vi "Main.vi"() -> ()   [LabVIEW 2021]
uses:
  controls/UI Data.ctl
  controls/ID.ctl
  controls/TCP states.ctl
  169f6d76-e22e-422a-8878-d2a9cb751e73.vi
  6a9415bc-3281-45d9-a9d8-b5f40684fea4.vi
  904bcb0e-ec7b-4b25-8705-34aa29b38f14.vi
  fb36bc3e-c328-4c18-9bea-3fff38157571.vi
  34653ac8-04e4-4dac-97e9-0b17219b7a3c.vi
  4f2ca51b-55f9-45ce-8b7e-e77bf4893014.vi
  ef0f1724-a7e1-494b-ab43-6d28ffb4e330.vi
  49fa5557-646f-45f4-af6f-6dd531291f5f.vi
  d94f9ece-38ec-4846-8ebf-07454e2bacb2.vi
panel:
  out "Response":string
  out "DS":bool
  out "WA":bool
  out "WC":bool
  in  "Stop":bool
  in  "My App path":path=path "c:/My App"
  in  "Reboot":bool
  out "PWR":bool
  out "WS":bool
  out "DC":bool
  out "SM":bool
  out "Commands":string[][](array[string])
  in  "Config path":path=path "C:/Users/ken_X/Documents/LabVIEW projects/Project-B/settings/config.xls"
  in  "Version path":path=path "C:/4.9.12.6034"
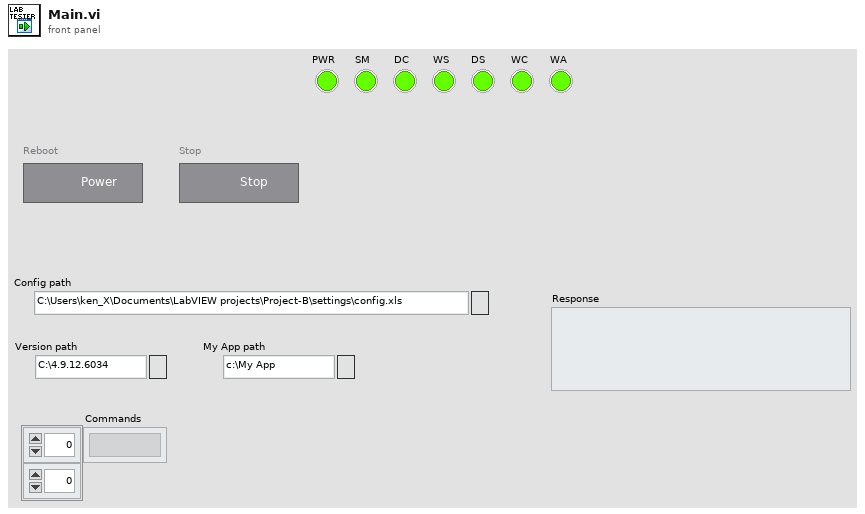
[diagram p1: front panel]
types:
  T1 = typedef "UI Data.ctl" = cluster{"Config path":path, "Version path":path, "My App path":path, "Racks":u16}
  T2 = cluster{"accent s color":u32, "accent s color":u32}
  T3 = typedef "ID.ctl" = enum16{"1 - PWR", "2 - SM", "3 - DC", "4 - DM", "5 - WS", "6 - DS", "7 - WC", "8 - WA", "9 - WM", "10 - DA", "11 - WH", "12 - DH"}
  T4 = typedef "TCP states.ctl" = string
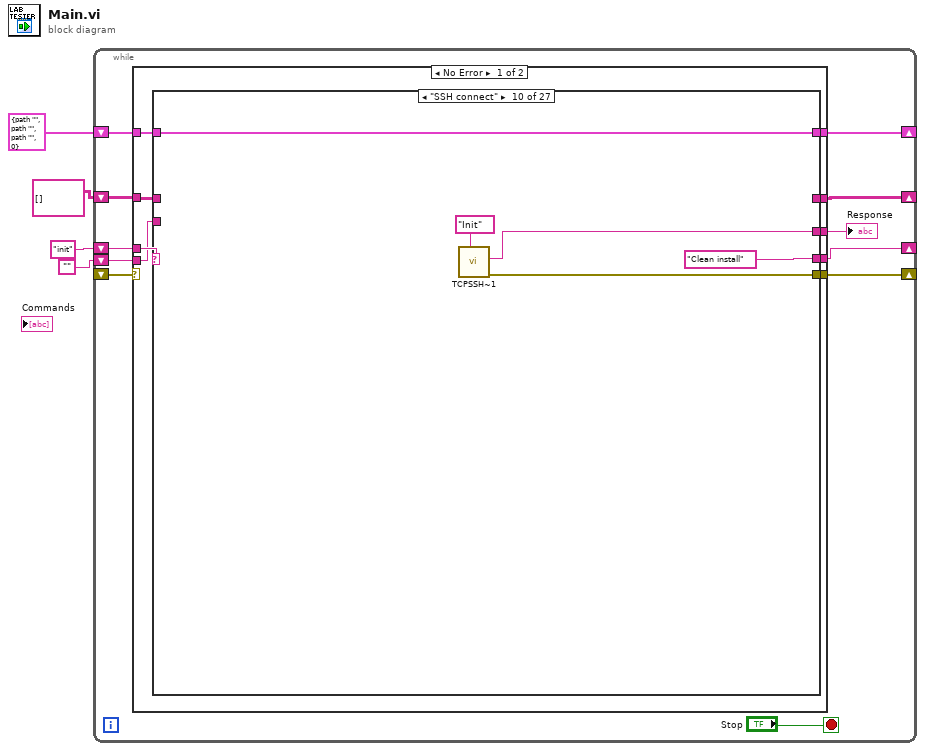
[diagram p0: block diagram]
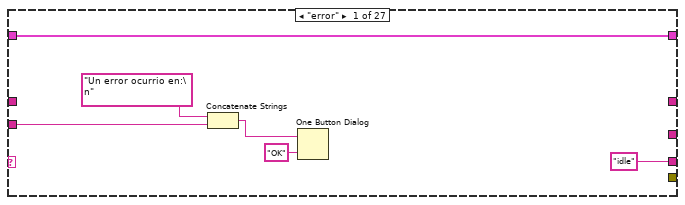
[diagram p2: hidden frame]
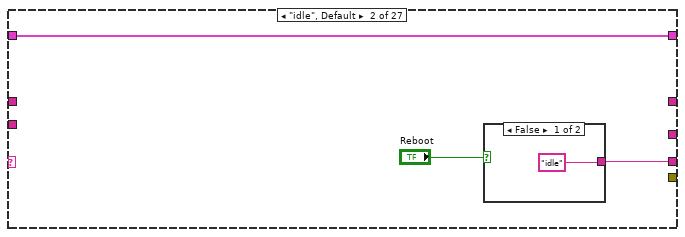
[diagram p3: hidden frame]
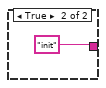
[diagram p4: hidden frame]
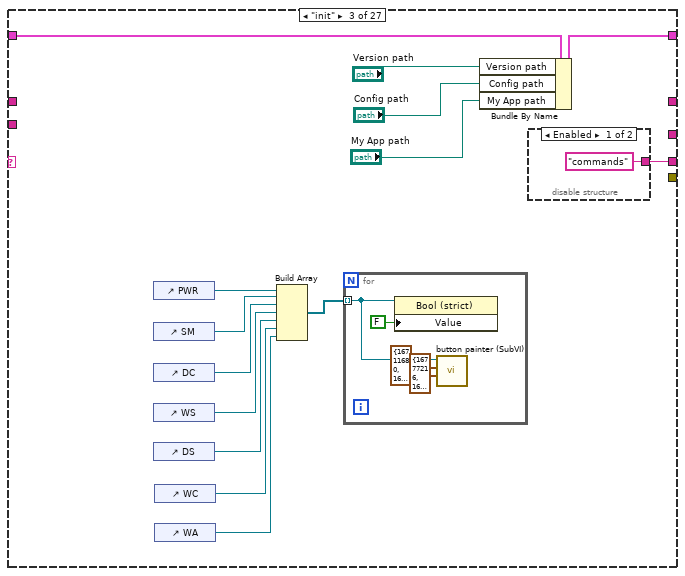
[diagram p5: hidden frame]
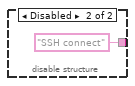
[diagram p6: hidden frame]
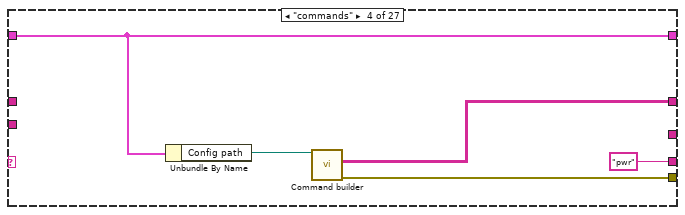
[diagram p7: hidden frame]
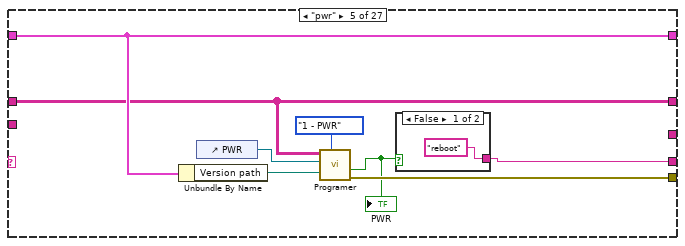
[diagram p8: hidden frame]
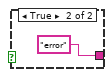
[diagram p9: hidden frame]
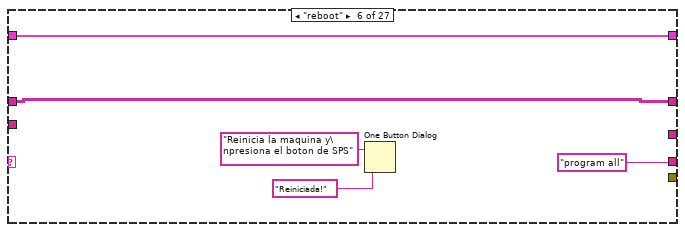
[diagram p10: hidden frame]
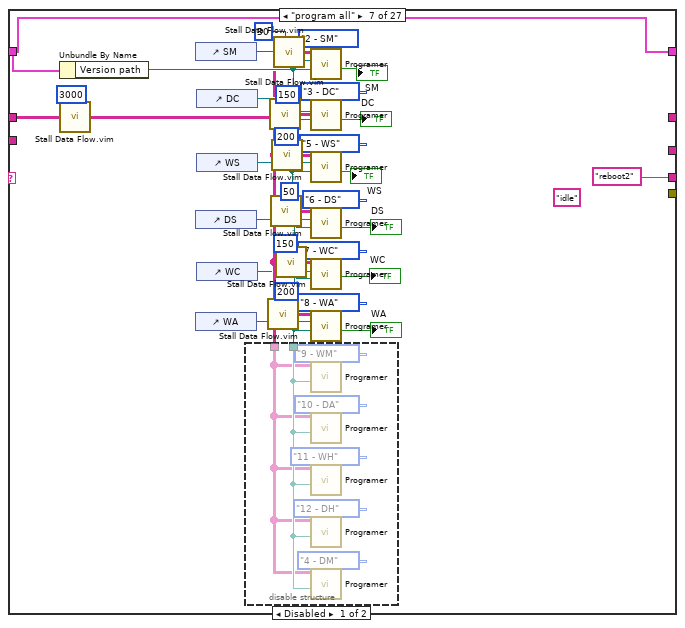
[diagram p11: hidden frame]
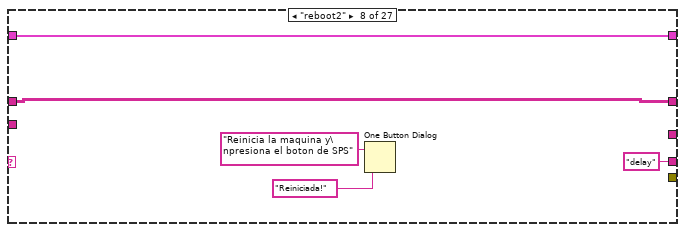
[diagram p13: hidden frame]
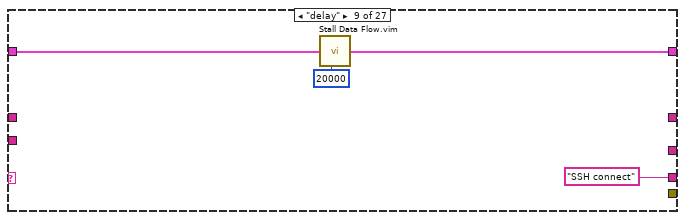
[diagram p14: hidden frame]
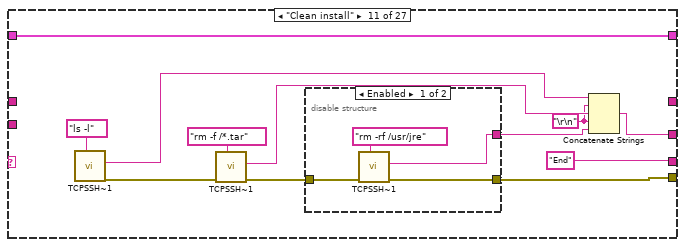
[diagram p15: hidden frame]
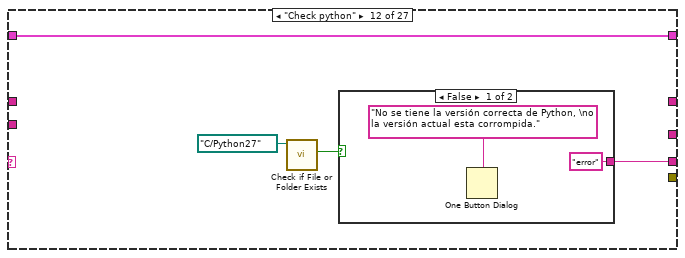
[diagram p17: hidden frame]
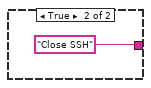
[diagram p18: hidden frame]
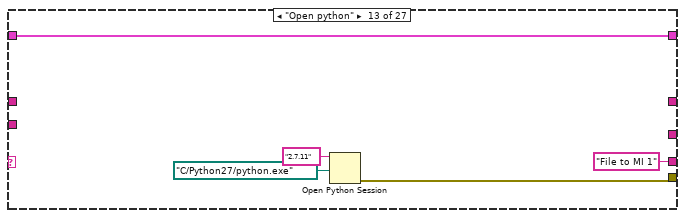
[diagram p19: hidden frame]
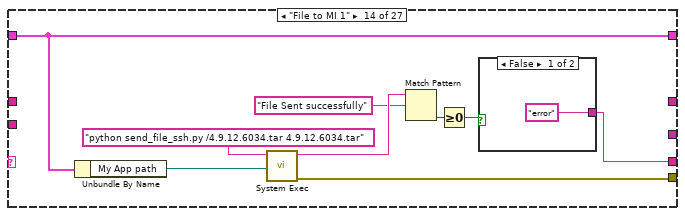
[diagram p20: hidden frame]
diagram:
  n1 = while {
    shift-right: [w13] -> _
    shift-left: T1 {"Config path"=path "", "Version path"=path "", "My App path"=path "", "Racks"=0} ("Cluster") -> [w14]
    shift-right: [w12] -> _
    shift-left: "init" -> [w15]
    shift-right: [w11] -> _
    shift-left: _ -> [w10]
    shift-right: [w9] -> _
    shift-left: string[][] [] ("Commands") -> [w8]
    shift-left: "" -> [w7]
    stop <- "Stop" stop-if-true
    n2 = case shown="No Error" w10 {
      selector: w10 -> [_ w296]
      tunnel: w15 -> [w24 _]
      tunnel: w14 -> [w23 _]
      tunnel: [w22 _] -> w13
      tunnel: [w21 "idle"] -> w12
      tunnel: [w20 _] -> w11
      tunnel: [w19 _] -> w9
      tunnel: w8 -> [w18 _]
      tunnel: w7 -> [w17 w295]
      tunnel: [w16 _] -> w5
      frame No Error {
        n3 = case shown="\"SSH connect\"" w24 {
          tunnel: w23 -> [w25 w33 w49 w57 w67 w71 w110 w120 w127 w129 w141 w153 w161 w164 w175 w189 w203 w207 w212 w227 w231 w241 w253 w259 w266 w290 w293]
          tunnel: [w25 w33 w48 w57 w67 w71 w110 w120 w125 w129 w141 w153 w161 w164 w175 w189 w203 w207 w212 w227 w231 w241 w253 w259 w265 w290 w293] -> w22
          tunnel: ["idle" w31 w47 "pwr" w62 "program all" "reboot2" "delay" "SSH connect" "Clean install" "End" w150 "File to MI 1" w165 w173 "Kill all" "Copy rootfs" "Sync" w208 "Telnet" "Search Data" w232 w244 "Check racks" w260 "End" "idle"] -> w21
          tunnel: [_ _ _ w60 w66 _ _ _ _ w131 w142 _ w158 w162 w177 w185 w192 w205 w209 w221 w229 w233 w245 w257 w263 w289 _] -> w20
          tunnel: [_ _ _ w58 w65 w72 _ w121 _ _ _ _ _ _ _ _ _ _ _ _ _ _ _ _ _ _ _] -> w19
          tunnel: w18 -> [_ _ _ _ w65 w72 w107 w121 _ _ _ _ _ _ _ _ _ _ _ _ _ _ _ _ _ _ _]
          tunnel: w17 -> [w29 _ _ _ _ _ _ _ _ _ _ _ _ _ _ _ _ _ _ _ _ _ _ _ _ _ _]
          tunnel: [_ _ _ _ _ _ _ _ _ w128 w138 _ _ _ _ _ _ _ _ _ _ _ _ _ _ _ _] -> w16
          frame "error" {
            n4 = Concatenate Strings("Un error ocurrio en:\n" ("string"), w29) -> (w28:string)
            n5 = One Button Dialog(message=w28, button name ("OK")="OK") -> ()  [unwired: 1 out]
          }
          frame "idle", Default {
            n6 = case shown="False" "Reboot" {
              tunnel: ["idle" "init"] -> w31
              frame False {
              }
              frame True {
              }
            }
          }
          frame "init" {
            n7 = control-ref of="PWR"() -> (w43:refnum<vi>)
            n8 = control-ref of="SM"() -> (w42:refnum<vi>)
            n9 = control-ref of="DC"() -> (w41:refnum<vi>)
            n10 = control-ref of="WS"() -> (w40:refnum<vi>)
            n11 = control-ref of="DS"() -> (w38:refnum<vi>)
            n12 = control-ref of="WC"() -> (w37:refnum<vi>)
            n13 = control-ref of="WA"() -> (w36:refnum<vi>)
            n14 = Build Array(w43, w42, w41, w40, w38, w37, w36) -> (w39:refnum<vi>[])
            n15 = for {
              tunnel: w39 -> [w54] mode=indexing
              n16 = property class="Bool (strict)"(reference=w54, "Value"=FALSE) -> ()  [unwired: 1 in, 2 out]
              n17 = call "button painter (SubVI).vi"("Off state"=cluster{"accent color":u32, "accent color":u32} {"accent color"=16777216, "accent color"=16777216}, "On state"=T2 {"accent s color"=16711680, "accent s color"=16711680}, "Button ref in"=w54) -> ()  [unwired: 9 in]
            }
            n18 = Bundle By Name(cluster=w49, "Version path"="Version path", "Config path"="Config path", "My App path"="My App path") -> (w48:T1)
            n19 = disable-structure shown="Enabled" {
              disable-tunnel: ["commands" "SSH connect"] -> w47
              frame Enabled {
              }
              frame Disabled {
              }
            }
          }
          frame "commands" {
            n20 = Unbundle By Name(w57) -> ("Config path"=w56:path)
            n21 = call "Command builder.vi"("Config path"=w56) -> ("error out"=w60:errorcluster, "Commands"=w58:string[][])  [unwired: 9 in]
          }
          frame "pwr" {
            n22 = Unbundle By Name(w67) -> ("Version path"=w63:path)
            n23 = control-ref of="PWR"() -> (w61:refnum<vi>)
            n24 = call "Programer.vi"("ID"=ID."1 - PWR", "version path"=w63, "Bool Ref"=w61, "Commands"=w65) -> ("error out"=w66:errorcluster, "error?"=w64:bool)  [unwired: 5 in, 1 out]
            "PWR" <- w64
            n25 = case shown="False" w64 {
              tunnel: ["reboot" "error"] -> w62
              frame False {
              }
              frame True {
              }
            }
          }
          frame "reboot" {
            n26 = One Button Dialog(message="Reinicia la maquina y\npresiona el boton de SPS", button name ("OK")="Reiniciada!") -> ()  [unwired: 1 out]
          }
          frame "program all" {
            (unwired) "idle"
            n27 = Unbundle By Name(w110) -> ("Version path"=w105:path)
            n28 = call "Stall Data Flow.vim"("value in"=w107, "milliseconds to wait"=u32 3000) -> ("value out"=w97:string[][])  [unwired: 1 out]
            n29 = control-ref of="SM"() -> (w104:refnum<vi>)
            n30 = control-ref of="DS"() -> (w92:refnum<vi>)
            n31 = control-ref of="WA"() -> (w90:refnum<vi>)
            n32 = control-ref of="DC"() -> (w103:refnum<vi>)
            n33 = control-ref of="WS"() -> (w102:refnum<vi>)
            n34 = control-ref of="WC"() -> (w91:refnum<vi>)
            n35 = disable-structure shown="Disabled" {
              disable-tunnel: w105 -> [w118 _]
              disable-tunnel: w97 -> [w117 _]
              frame Disabled {
                n36 = call "Programer.vi"("ID"=ID."9 - WM", "version path"=w118, "Commands"=w117) -> ()  [unwired: 6 in, 3 out]
                n37 = call "Programer.vi"("ID"=ID."10 - DA", "version path"=w118, "Commands"=w117) -> ()  [unwired: 6 in, 3 out]
                n38 = call "Programer.vi"("ID"=ID."11 - WH", "version path"=w118, "Commands"=w117) -> ()  [unwired: 6 in, 3 out]
                n39 = call "Programer.vi"("ID"=ID."12 - DH", "version path"=w118, "Commands"=w117) -> ()  [unwired: 6 in, 3 out]
                n40 = call "Programer.vi"("ID"=ID."4 - DM", "version path"=w118, "Commands"=w117) -> ()  [unwired: 6 in, 3 out]
              }
              frame Enabled {
              }
            }
            n41 = call "Stall Data Flow.vim"("value in"=w97, "milliseconds to wait"=u32 200) -> ("value out"=w78:string[][])  [unwired: 1 out]
            n42 = call "Stall Data Flow.vim"("value in"=w97, "milliseconds to wait"=u32 150) -> ("value out"=w86:string[][])  [unwired: 1 out]
            n43 = call "Stall Data Flow.vim"("value in"=w97, "milliseconds to wait"=u32 50) -> ("value out"=w82:string[][])  [unwired: 1 out]
            n44 = call "Stall Data Flow.vim"("value in"=w97, "milliseconds to wait"=u32 200) -> ("value out"=w84:string[][])  [unwired: 1 out]
            n45 = call "Stall Data Flow.vim"("value in"=w97, "milliseconds to wait"=u32 50) -> ("value out"=w99:string[][])  [unwired: 1 out]
            n46 = call "Stall Data Flow.vim"("value in"=w97, "milliseconds to wait"=u32 150) -> ("value out"=w80:string[][])  [unwired: 1 out]
            n47 = call "Programer.vi"("ID"=ID."2 - SM", "version path"=w105, "Bool Ref"=w104, "Commands"=w99) -> ("error?"=→"SM":bool)  [unwired: 5 in, 2 out]
            n48 = call "Programer.vi"("ID"=ID."3 - DC", "version path"=w105, "Bool Ref"=w103, "Commands"=w86) -> ("error?"=→"DC":bool)  [unwired: 5 in, 2 out]
            n49 = call "Programer.vi"("ID"=ID."5 - WS", "version path"=w105, "Bool Ref"=w102, "Commands"=w84) -> ("error?"=→"WS":bool)  [unwired: 5 in, 2 out]
            n50 = call "Programer.vi"("ID"=ID."6 - DS", "version path"=w105, "Bool Ref"=w92, "Commands"=w82) -> ("error?"=→"DS":bool)  [unwired: 5 in, 2 out]
            n51 = call "Programer.vi"("ID"=ID."7 - WC", "version path"=w105, "Bool Ref"=w91, "Commands"=w80) -> ("error?"=→"WC":bool)  [unwired: 5 in, 2 out]
            n52 = call "Programer.vi"("ID"=ID."8 - WA", "version path"=w105, "Bool Ref"=w90, "Commands"=w78) -> ("error?"=→"WA":bool)  [unwired: 5 in, 2 out]
          }
          frame "reboot2" {
            n53 = One Button Dialog(message="Reinicia la maquina y\npresiona el boton de SPS", button name ("OK")="Reiniciada!") -> ()  [unwired: 1 out]
          }
          frame "delay" {
            n54 = call "Stall Data Flow.vim"("value in"=w127, "milliseconds to wait"=u32 20000) -> ("value out"=w125:T1)  [unwired: 1 out]
          }
          frame "SSH connect" {
            n55 = call "TCPSSH~1.VI"("States"=T4 "Init") -> ("Error  Out"=w131:errorcluster, "Response"=w128:string)  [unwired: 8 in]
          }
          frame "Clean install" {
            w134 = "\r\n"
            n56 = call "TCPSSH~1.VI"("States"=T4 "ls -l") -> ("Error  Out"=w135:errorcluster, "Response"=w133:string)  [unwired: 8 in]
            n57 = call "TCPSSH~1.VI"("States"=T4 "rm -f /*.tar", "Error In"=w135) -> ("Error  Out"=w144:errorcluster, "Response"=w140:string)  [unwired: 7 in]
            n58 = disable-structure shown="Enabled" {
              disable-tunnel: w144 -> [w148 w149]
              disable-tunnel: [w146 w149] -> w142
              disable-tunnel: [w145 _] -> w139
              frame Enabled {
                n59 = call "TCPSSH~1.VI"("States"=T4 "rm -rf /usr/jre", "Error In"=w148) -> ("Error  Out"=w146:errorcluster, "Response"=w145:string)  [unwired: 7 in]
              }
              frame Disabled {
              }
            }
            n60 = Concatenate Strings(w133, w134, w140, w134, w139) -> (w138:string)
          }
          frame "Check python" {
            n61 = call <vilib>:"Check if File or Folder Exists.vi"("path"=path "C:/Python27") -> ("file or folder exists?"=w151:bool)  [unwired: 8 in, 2 out]
            n62 = case shown="False" w151 {
              tunnel: ["error" "Close SSH"] -> w150
              frame False {
                n63 = One Button Dialog(message="No se tiene la versión correcta de Python, \no la versión actual esta corrompida.") -> ()  [unwired: 1 in, 1 out]
              }
              frame True {
              }
            }
          }
          frame "Open python" {
            n64 = Open Python Session(python version="2.7.11" ("Python version"), python path=path "C:/Python27/python.exe" ("Python path")) -> (error out=w158:errorcluster)  [unwired: 1 in, 1 out]
          }
          frame "File to MI 1" {
            n65 = Unbundle By Name(w164) -> ("My App path"=w163:path)
            n66 = call <vilib>:"System Exec.vi"("working directory"=w163, "command line"="python send_file_ssh.py /4.9.12.6034.tar 4.9.12.6034.tar") -> ("error out"=w162:errorcluster, "standard output"=w169:string)  [unwired: 6 in, 2 out]
            n67 = Match Pattern(string=w169, regular expression="File Sent successfully") -> (offset past match=w167:i32)  [unwired: 1 in, 3 out]
            n68 = Greater Or Equal To 0?(x=w167) -> (x >= 0?=w166:bool)
            n69 = case shown="False" w166 {
              tunnel: ["error" "End"] -> w165
              frame False {
              }
              frame True {
                (unwired) "File to MI 2"
              }
            }
          }
          frame "File to MI 2" {
            n70 = Unbundle By Name(w175) -> ("My App path"=w174:path)
            n71 = call <vilib>:"System Exec.vi"("working directory"=w174, "command line"="send_file_to_MI_ssh.bat /jre.tar.gz jre.tar.gz") -> ("error out"=w177:errorcluster, "standard output"=w181:string)  [unwired: 6 in, 2 out]
            n72 = Match Pattern(string=w181, regular expression="File Sent successfully") -> (offset past match=w179:i32)  [unwired: 1 in, 3 out]
            n73 = Greater Or Equal To 0?(x=w179) -> (x >= 0?=w178:bool)
            n74 = case shown="True" w178 {
              tunnel: ["error" "Send tars"] -> w173
              frame False {
              }
              frame True {
              }
            }
          }
          frame "Send tars" {
            n75 = call "TCPSSH~1.VI"("States"=T4 "tar -xvf 4.9.12.6034.tar") -> ("Error  Out"=w188:errorcluster)  [unwired: 8 in, 1 out]
            n76 = call "TCPSSH~1.VI"("States"=T4 "tar -xvf jre.tar.gz -C /usr", "Error In"=w188) -> ("Error  Out"=w185:errorcluster)  [unwired: 7 in, 1 out]
          }
          frame "Kill all" {
            n77 = call "TCPSSH~1.VI"("States"=T4 "rm -f /*.tar") -> ("Error  Out"=w194:errorcluster)  [unwired: 8 in, 1 out]
            n78 = call "TCPSSH~1.VI"("States"=T4 "rm -f /*.gz", "Error In"=w194) -> ("Error  Out"=w196:errorcluster)  [unwired: 7 in, 1 out]
            n79 = call "TCPSSH~1.VI"("States"=T4 "killall DataProcessor.exe", "Error In"=w196) -> ("Error  Out"=w197:errorcluster)  [unwired: 7 in, 1 out]
            n80 = call "TCPSSH~1.VI"("States"=T4 "killall WIFIAgent.exe", "Error In"=w197) -> ("Error  Out"=w199:errorcluster)  [unwired: 7 in, 1 out]
            n81 = call "TCPSSH~1.VI"("States"=T4 "killall java", "Error In"=w199) -> ("Error  Out"=w201:errorcluster)  [unwired: 7 in, 1 out]
            n82 = call "TCPSSH~1.VI"("States"=T4 "killall MonitorDaemon.exe", "Error In"=w201) -> ("Error  Out"=w192:errorcluster)  [unwired: 7 in, 1 out]
          }
          frame "Copy rootfs" {
            n83 = call "TCPSSH~1.VI"("States"=T4 "cp -rf rootfs/* /") -> ("Error  Out"=w205:errorcluster)  [unwired: 8 in, 1 out]
          }
          frame "Sync" {
            n84 = flat-sequence {
              tunnel: [w213] -> w211
              tunnel: w211 -> [w217]
              tunnel: [w216] -> w210
              tunnel: [w219] -> w209
              tunnel: w210 -> [w219]
              tunnel: ["SED"] -> w208
              frame #0 {
                n85 = call "TCPSSH~1.VI"("States"=T4 "sync") -> ("Error  Out"=w213:errorcluster)  [unwired: 8 in, 1 out]
              }
              frame #1 {
                n86 = call "Stall Data Flow.vim"("value in"=w217, "milliseconds to wait"=u32 3000) -> ("value out"=w216:errorcluster)  [unwired: 1 out]
              }
              frame #2 {
              }
            }
          }
          frame "SED" {
            n87 = call "TCPSSH~1.VI"("States"=T4 "cd hdplus") -> ("Error  Out"=w224:errorcluster)  [unwired: 8 in, 1 out]
            n88 = call "TCPSSH~1.VI"("States"=T4 "sed -i", "Error In"=w224) -> ("Error  Out"=w226:errorcluster)  [unwired: 7 in, 1 out]
            n89 = call "TCPSSH~1.VI"("States"=T4 "cat /hdplus/tablo.conf", "Error In"=w226) -> ("Error  Out"=w221:errorcluster)  [unwired: 7 in, 1 out]
          }
          frame "Telnet" {
            n90 = call "TCPSSH~1.VI"("States"=T4 "script/disableTelnet") -> ("Error  Out"=w229:errorcluster)  [unwired: 8 in, 1 out]
          }
          frame "Search Data" {
            n91 = call "TCPSSH~1.VI"("States"=T4 "ls -l") -> ("Error  Out"=w235:errorcluster)  [unwired: 8 in, 1 out]
            n92 = call "TCPSSH~1.VI"("States"=T4 "Read", "Error In"=w235) -> ("Error  Out"=w233:errorcluster, "Response"=w240:string)  [unwired: 7 in]
            n93 = Match Pattern(string=w240, regular expression="DataProcessor.exe") -> (offset past match=w237:i32)  [unwired: 1 in, 3 out]
            n94 = Greater Or Equal To 0?(x=w237) -> (x >= 0?=w238:bool)
            n95 = case shown="True" w238 {
              tunnel: ["error" "Search Java"] -> w232
              frame False {
              }
              frame True {
              }
            }
          }
          frame "Search Java" {
            n96 = call "TCPSSH~1.VI"("States"=T4 "/usr/jre/bin/java -version") -> ("Error  Out"=w247:errorcluster)  [unwired: 8 in, 1 out]
            n97 = call "TCPSSH~1.VI"("States"=T4 "Read", "Error In"=w247) -> ("Error  Out"=w245:errorcluster, "Response"=w252:string)  [unwired: 7 in]
            n98 = Match Pattern(string=w252, regular expression="1.8.0-b132") -> (offset past match=w249:i32)  [unwired: 1 in, 3 out]
            n99 = Greater Or Equal To 0?(x=w249) -> (x >= 0?=w250:bool)
            n100 = case shown="True" w250 {
              tunnel: ["error" "Dev"] -> w244
              frame False {
              }
              frame True {
              }
            }
          }
          frame "Dev" {
            n101 = call "TCPSSH~1.VI"("States"=T4 "cd /dev") -> ("Error  Out"=w257:errorcluster)  [unwired: 8 in, 1 out]
          }
          frame "Check racks" {
            n102 = Unbundle By Name(w266) -> ("Racks"=w261:u16)
            n103 = Equal To 0?(x=w261) -> (x = 0?=w262:bool)
            n104 = case shown="False" w262 {
              tunnel: w261 -> [w274 w285]
              tunnel: [w273 w285] -> w264
              tunnel: [w268 _] -> w263
              tunnel: [w267 "End"] -> w260
              frame False {
                n105 = call "TCPSSH~1.VI"("States"=T4 "ls sd* -l") -> ("Error  Out"=w272:errorcluster)  [unwired: 8 in, 1 out]
                n106 = call "TCPSSH~1.VI"("States"=T4 "Read", "Error In"=w272) -> ("Error  Out"=w268:errorcluster, "Response"=w269:string)  [unwired: 7 in]
                n107 = call "string pattern counter.vi"("pattern"="root", "string"=w269) -> ("Numeric"=w277:i32)  [unwired: 9 in]
                n108 = Multiply(x=w274, y=2) -> (x*y=w281:i32)
                n109 = Equal?(x=w281, y=w277) -> (x = y?=w276:bool)
                n110 = Format Into String(format string="Quite una de las %d unidades montadas", w274) -> (resulting string=w275:string)  [unwired: 2 in, 1 out]
                n111 = case shown="True" w276 {
                  tunnel: w275 -> [_ w284]
                  tunnel: ["error" "Check racks"] -> w267
                  frame False {
                  }
                  frame True {
                    n112 = One Button Dialog(message=w284) -> ()  [unwired: 1 in, 1 out]
                  }
                }
                n113 = Decrement(x=w274) -> (x-1=w273:u16)
              }
              frame True {
              }
            }
            n114 = Bundle By Name(cluster=w266, "Racks"=w264) -> (w265:T1)
          }
          frame "Close SSH" {
            n115 = call "TCPSSH~1.VI"("States"=T4 "Close") -> ("Error  Out"=w289:errorcluster)  [unwired: 8 in, 1 out]
          }
          frame "End" {
            n116 = One Button Dialog(message="Proceso terminado!!!") -> ()  [unwired: 1 in, 1 out]
          }
        }
      }
      frame Error {
        n117 = call <vilib>:"Simple Error Handler.vi"("error source (\" \")"=w295, "error in (no error)"=w296) -> ("error out"=w294:errorcluster)  [unwired: 3 in, 4 out]
        n118 = call <vilib>:"Clear Errors.vi"("error in (no error)"=w294) -> ()  [unwired: 5 in, 2 out]
      }
    }
    "Response" <- w5
  }
